vi "Shift Cursor.vi"(6 "chip select  (1st chip)":enum16{"1st chip", "2nd chip"}(ring), 8 "error in (no error)":errorcluster, 10 "direction":enum16{"left", "right"}(ring), 11 "HD44780 in":refnum<class "HD44780.lvclass">) -> (0 "error out":errorcluster, 3 "HD44780 out":refnum<class "HD44780.lvclass">)   [LabVIEW 2017, in "HD44780.lvclass"]
uses:
  HD44780.lvclass
  HD44780.lvclass/HD44780.ctl
  Common/HD44780 Common.lvlib
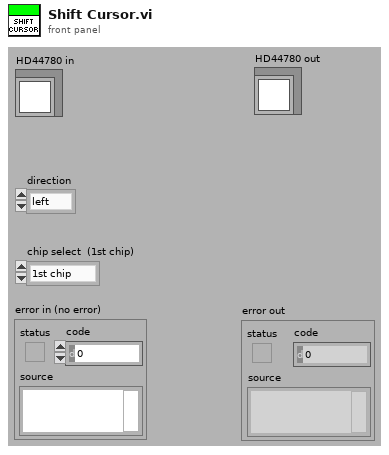
[diagram p1: front panel]
types:
  T1 = typedef "HD44780 Common.lvlib/cluster of class private data.ctl" = cluster{"FPGA VI Reference":refnum<k20>, "device index":i8, "screen size":T2, "font size":T3, "auto wrap":bool, "alignment":T4, "number of line":T5, "shift 0":i8, "entry mode 0":T6, "shift 1":i8, "entry mode 1":T6}
  T2 = typedef "HD44780 Common.lvlib/screen size.ctl" = enum8{"8x1", "8x2", "12x4", "16x1", "16x2", "16x4", "20x1", "20x2", "20x4", "24x1", "24x2", "40x2", "40x4"}
  T3 = typedef "HD44780 Common.lvlib/font size.ctl" = enum8{"5x8", "5x10"}
  T4 = typedef "HD44780 Common.lvlib/alignment.ctl" = enum16{"None", "Left", "Center", "Right"}
  T5 = typedef "HD44780 Common.lvlib/line number.ctl" = enum8{"1 line", "2 lines"}
  T6 = typedef "HD44780 Common.lvlib/entry mode.ctl" = enum8{"increment & no shift", "increment & shift", "decrement & no shift", "decrement & shift"}
  T7 = cluster{"FPGA VI Reference":refnum<k20>, "device index":i8, "screen size":enum8{"8x1", "8x2", "12x4", "16x1", "16x2", "16x4", "20x1", "20x2", "20x4", "24x1", "24x2", "40x2", "40x4"}, "font size":enum8{"5x8", "5x10"}, "auto wrap":bool, "alignment":enum16{"None", "Left", "Center", "Right"}, "number of line":enum8{"1 line", "2 lines"}, "shift 0":i8, "entry mode 0":enum8{"increment & no shift", "increment & shift", "decrement & no shift", "decrement & shift"}, "shift 1":i8, "entry mode 1":enum8{"increment & no shift", "increment & shift", "decrement & no shift", "decrement & shift"}}
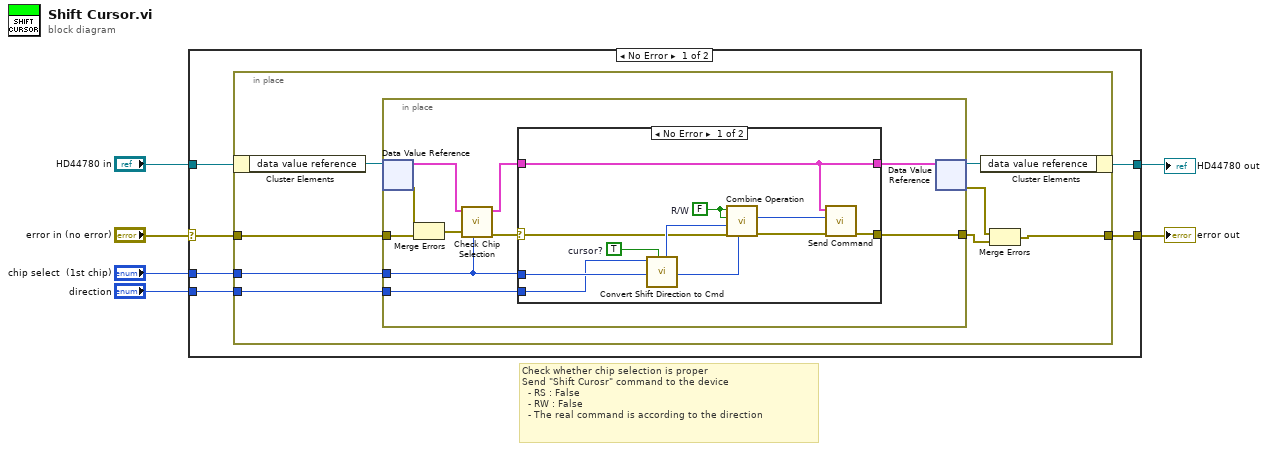
[diagram p0: block diagram]
diagram:
  # "Check whether chip selection is proper\nSend \"Shift Curosr\" command to the device\n  - RS : False\n  - RW : False\n  - The real command is according to the direction"
  n1 = case shown="No Error" "error in (no error)" {
    selector: "error in (no error)" -> [w8 w43]
    tunnel: [w12 w43] -> w6
    tunnel: "chip select  (1st chip)" -> [w11 _]
    tunnel: "HD44780 in" -> [w10 w44]
    tunnel: [w9 w44] -> w2
    tunnel: "direction" -> [w7 _]
    frame No Error {
      n2 = in-place {
        in-place-border: [w16] -> w12
        in-place-border: w11 -> [w20]
        in-place-border: w8 -> [w15]
        in-place-border: w7 -> [w13]
        n3 = in-place-cluster #1(w10) -> ("data value reference"=w19:refnum<data-value>)
        n4 = in-place {
          in-place-border: w20 -> [w25]
          in-place-border: w15 -> [w27]
          in-place-border: [w22] -> w14
          in-place-border: w13 -> [w21]
          n5 = in-place-dvr #2(w19) -> (w30:T1, w28:errorcluster)
          n6 = Merge Errors(w28, w27) -> (w23:errorcluster)
          n7 = call "Check Chip Selection.vi"("chip select"=w25, "error in (no error)"=w23, "cluster of private data in"=w30) -> ("error out"=w24:errorcluster, "cluster of private data out"=w29:T7)  [unwired: 7 in]
          n8 = case shown="No Error" w24 {
            selector: w24 -> [w33 w41]
            tunnel: w29 -> [w34 w42]
            tunnel: w25 -> [w35 _]
            tunnel: [w34 w42] -> w26
            tunnel: [w32 w41] -> w22
            tunnel: w21 -> [w31 _]
            frame No Error {
              w38 = TRUE  # cursor?
              w40 = FALSE  # R/W
              n9 = call "Convert Shift Direction to Cmd.vi"("cursor?"=w38, "direction"=w31) -> ("LCD data/cmd"=w39:u8)  [unwired: 9 in]
              n10 = call "Combine Operation.vi"("chip select  (1st chip)"=w35, "error in (no error)"=w33, "cmd/data"=w39, "RS"=w40, "R/W"=w40) -> ("error out"=w37:errorcluster, "output"=w36:u32)  [unwired: 5 in]
              n11 = call "Send Command.vi"("error in (no error)"=w37, "operation"=w36, "cluster of private data in"=w34) -> ("error out"=w32:errorcluster)  [unwired: 6 in, 2 out]
            }
            frame Error {
            }
          }
          n12 = in-place-dvr #2(w26) -> (w18:refnum<data-value>, w17:errorcluster)
        }
        n13 = in-place-cluster #1("data value reference"=w18) -> (w9:refnum<class "HD44780.lvclass">)
        n14 = Merge Errors(w17, w14) -> (w16:errorcluster)
      }
    }
    frame Error {
    }
  }
  "error out" <- w6
  "HD44780 out" <- w2
